vi "Write PID Temp Setpoint.vi"(8 "error in (no error)":errorcluster, 10 "PID Temp Setpoint":dbl[unit], 11 "Temperature Controller in":refnum<class "Temperature Controller.lvclass">) -> (0 "error out":errorcluster, 3 "Temperature Controller out":refnum<class "Temperature Controller.lvclass">)   [LabVIEW 2015, in "Temperature Controller.lvclass"]
uses:
  Temperature Controller.lvclass
  Temperature Controller.lvclass/Temperature Controller.ctl
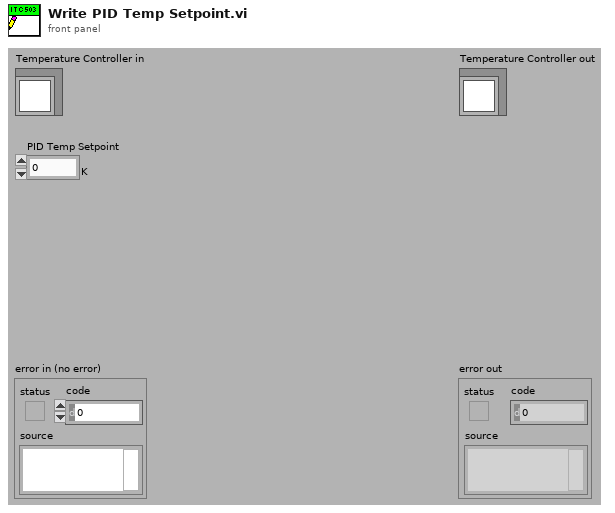
[diagram p1: front panel]
types:
  T1 = typedef "ITCIO.ctl" = cluster{"Address":T2, "Version":T3, "Ch 1 dec places":i16, "Ch 2 dec places":i16, "Ch 3 dec places":i16, "Ch1 Name":string, "Ch2 Name":string, "Ch3 Name":string}
  T2 = typedef "OxfordAddress.ctl" = cluster{"Com Port":i32, "ISOBUS Address":i32, "GPIB Address":i16, "Communication":enum16{"RS232", "ISOBUS", "GPIB", "Gateway"}}
  T3 = typedef "ITCVersion.ctl" = enum16{"ITC502", "ITC503", "ITC601"}
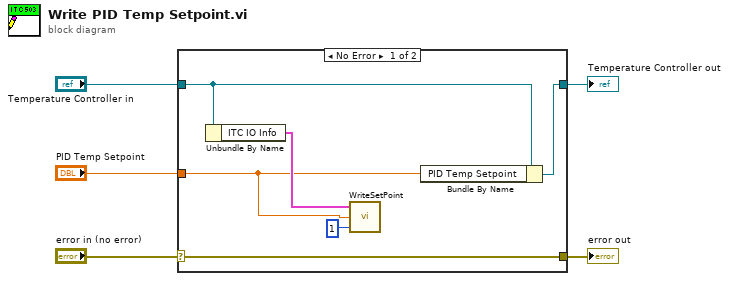
[diagram p0: block diagram]
diagram:
  n1 = case shown="No Error" "error in (no error)" {
    selector: "error in (no error)" -> [w11 w12]
    tunnel: [w11 w12] -> w4
    tunnel: [w10 w13] -> w2
    tunnel: "Temperature Controller in" -> [w8 w13]
    tunnel: "PID Temp Setpoint" -> [w6 _]
    frame No Error {
      n2 = Unbundle By Name(w8) -> ("ITC IO Info"=w7:T1)
      n3 = call "WriteSetPoint.vi"("Control Ch"=1, "Set point"=w6, "IO Info"=w7) -> ()  [unwired: 1 out]
      n4 = Bundle By Name(cluster=w8, "PID Temp Setpoint"=w6) -> (w10:refnum<class "Temperature Controller.lvclass">)
    }
    frame Error {
    }
  }
  "error out" <- w4
  "Temperature Controller out" <- w2
